vi "draw an ellipse.vi"(4 "ellipse factor":dbl=10.0, 6 "number of points":i32=20, 8 "curvature tensor IN":T3={"curvature Matrix"=[[3.0, 1.0], [1.0, 4.0]], "Eigenvalues"=[], "Eigenvectors"=[], "theta (rad)"=0.0+0.0i, "theta (deg)"=0.0+0.0i}, 10 "curvature Matrix IN":T1, 11 "center IN":cluster{"center x":dbl, "center Y":dbl}) -> (0 "curvature tensor OUT":T3={"curvature Matrix"=[[3.0, 1.0], [1.0, 4.0]], "Eigenvalues"=[4.618033988749895+0.0i, 2.381966011250105+0.0i], "Eigenvectors"=[[-0.8506508083520399+0.0i, -0.5257311121191335+0.0i], [0.5257311121191335+0.0i, -0.8506508083520399+0.0i]], "theta (rad)"=0.5535743588970453+0.0i, "theta (deg)"=31.717474411461012+0.0i}, 2 "curvature Matrix OUT":T1=[[3.0, 1.0], [1.0, 4.0]], 3 "ellipse OUT":cluster{"Array":dbl[], "Array":dbl[]})   [LabVIEW 2020]
uses:
  <vilib>/Analysis/Matrix/Datatypes/RealMatrix.ctl
  <vilib>/Analysis/Matrix/Datatypes/ComplexMatrix.ctl
  <vilib>/Analysis/7linalg.llb/Eigenvalue and Vectors Output Option.ctl
  array -- bilinear regression 2D.ctl
  <vilib>/Analysis/coordinate.llb/2D Cartesian Coordinate Rotation (Array).vi
  generate linear region.vi
  <vilib>/Analysis/7linalg.llb/Real Eigenvalues and Vectors.vi
  <vilib>/Analysis/Matrix/Numeric/Conversions/Matrix To Array - CM.vi
  <vilib>/Analysis/NI_AALPro.lvlib
  <vilib>/Analysis/Matrix/NI_Matrix.lvlib
panel:
  out "angle1":dbl=2.1243706856919418
  out "Plot: curvature":cluster{dbl[], dbl[]}(graph)
  out "z out":dbl[](array[numeric])
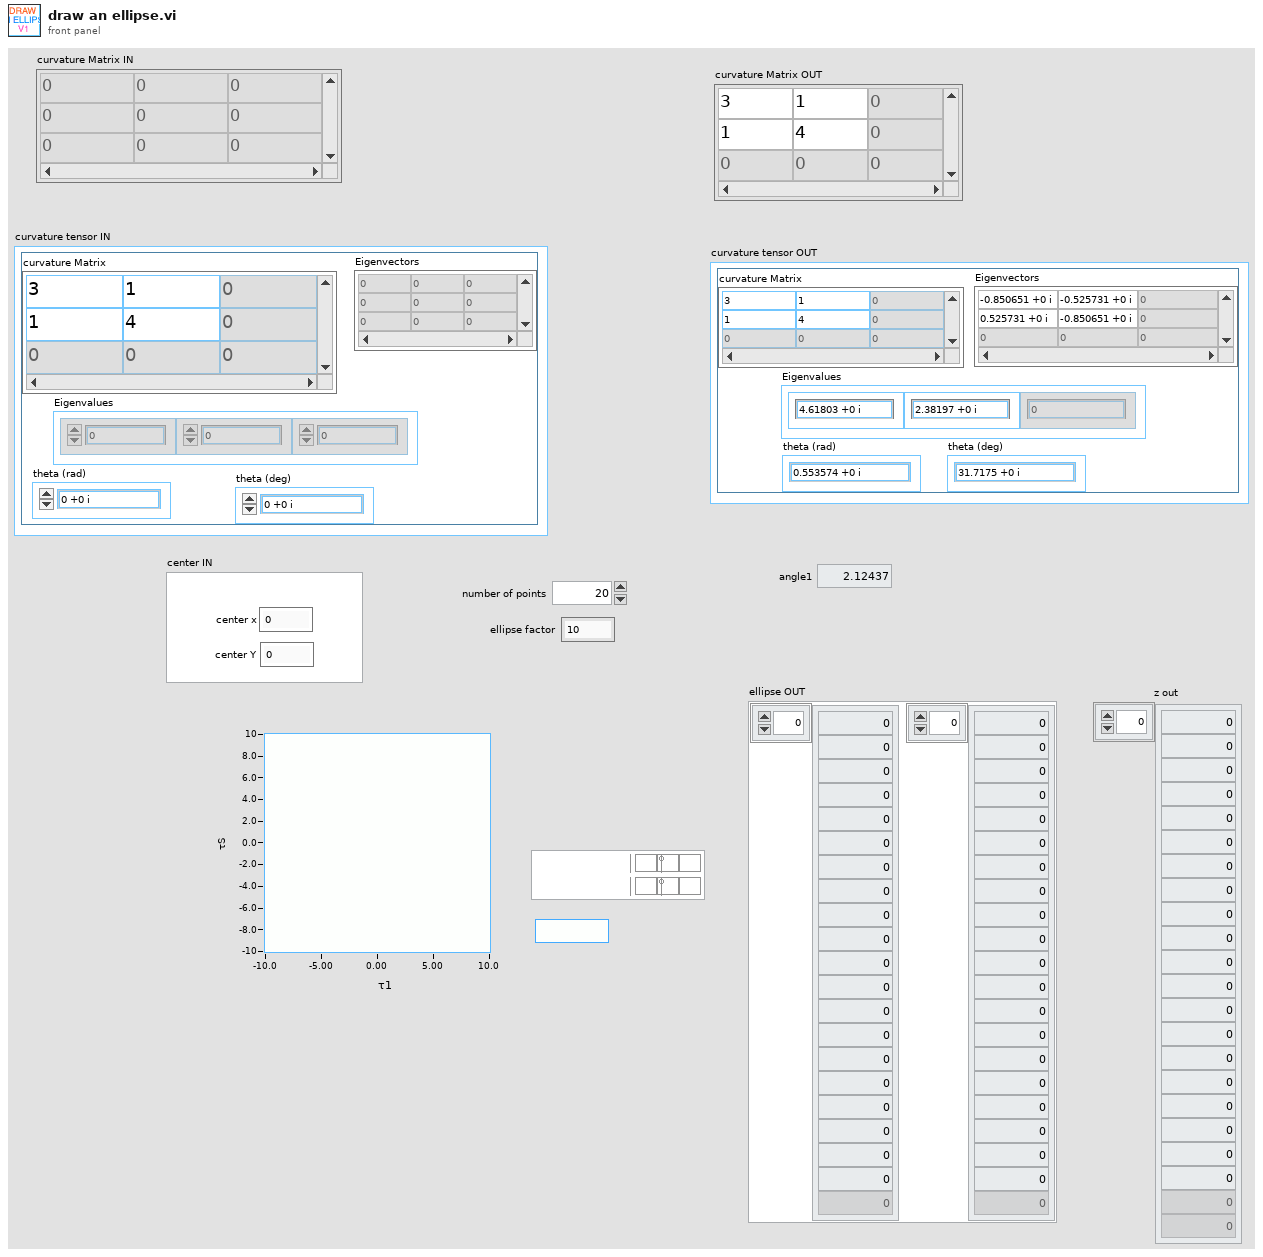
[diagram p1: front panel]
types:
  T1 = typedef "NI_Matrix.lvlib/RealMatrix.ctl" = dbl[][]
  T2 = typedef "NI_Matrix.lvlib/ComplexMatrix.ctl" = cdb[][]
  T3 = cluster{"curvature Matrix":T1, "Eigenvalues":cdb[], "Eigenvectors":T2, "theta (rad)":cdb, "theta (deg)":cdb}
  T4 = typedef "array -- bilinear regression 2D.ctl" = enum16{"1", "x", "y", "xx", "xy", "yy", "xxy", "xyy", "yyy", "xxx", "xxyy", "xyyy", "xxxy", "yyyy", "xxxx", "xxz", "xyz", "yyz", "xz", "yz", "z"}
  T5 = typedef "NI_AALPro.lvlib/Eigenvalue and Vectors Output Option.ctl" = i32
  T6 = cluster{"curvature Matrix":T1, dbl[], "Eigenvectors":T2, dbl, dbl}
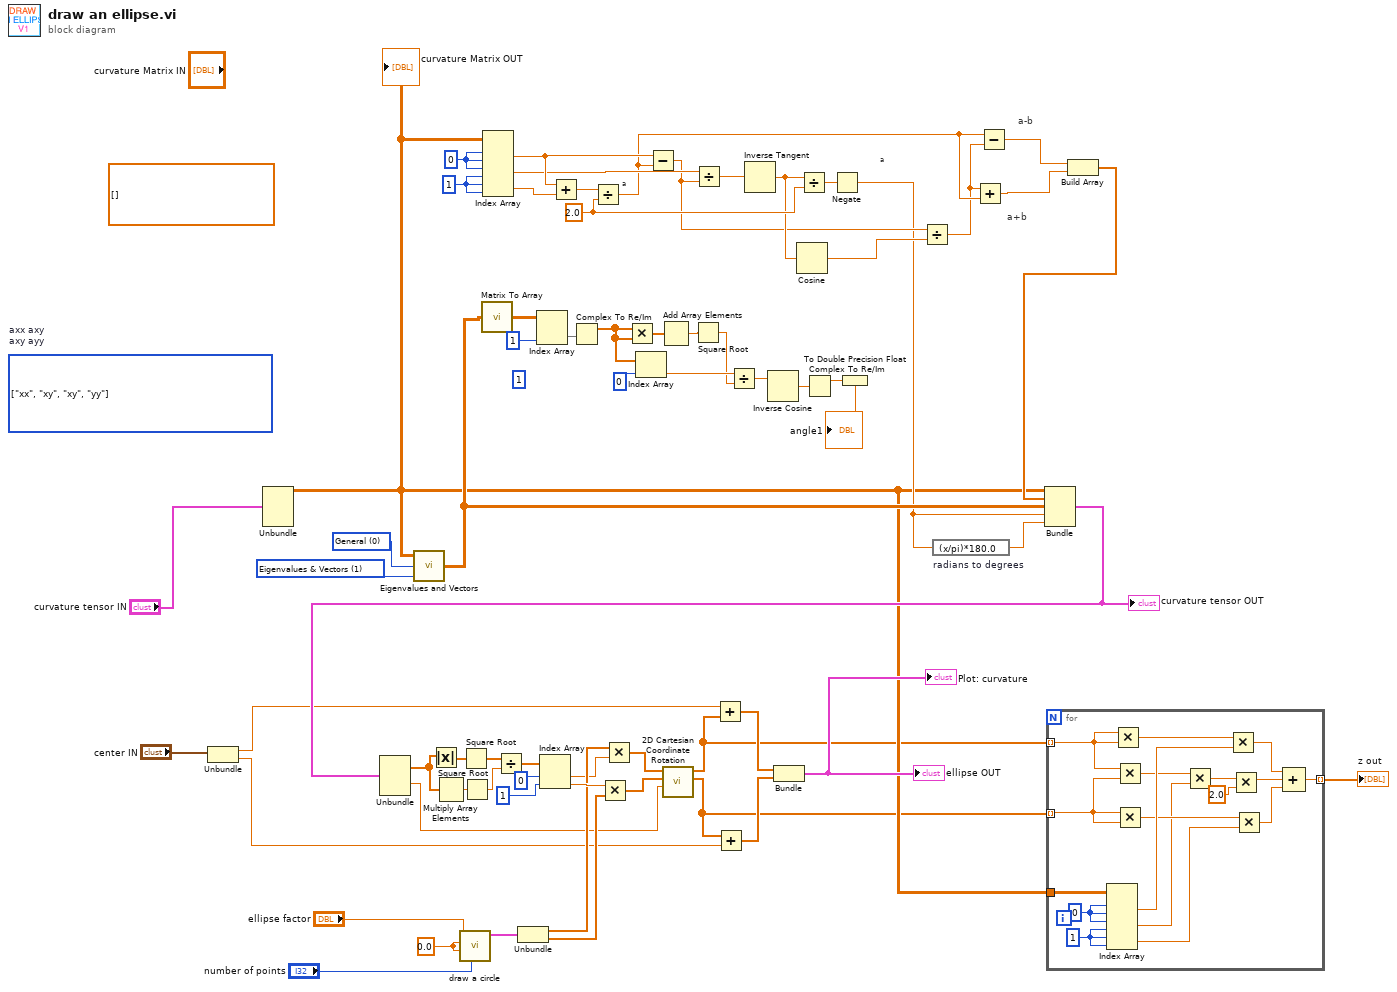
[diagram p0: block diagram]
diagram:
  (unwired) T1 [] ("curvature Matrix IN")
  w25 = 2.0 ("y")
  w30 = 1 ("index (row)")
  w31 = 0 ("index (row)")
  (unwired) T4[][] [[enum."xx", enum."xy"], [enum."xy", enum."yy"]] items=["1", "x", "y", "xx", "xy", "yy", "xxy", "xyy", "yyy", "xxx", "xxyy", "xyyy", "xxxy", "yyyy", "xxxx", "xxz", "xyz", "yyz", "xz", "yz", "z"]  # axx axy axy ayy
  (unwired) 1 ("length")
  w55 = T5 1 items=["Eigenvalues", "Eigenvalues & Vectors"] ("output option")
  w54 = 0 items=["General", "Symmetric"] ("matrix type")
  w58 = 0.0 ("center x")
  # "a-b"
  # "a+b"
  # "a"
  # "a"
  n1 = Unbundle("center IN") -> ("center x"=w4:dbl, "center Y"=w3:dbl)
  n2 = Unbundle("curvature tensor IN") -> ("curvature Matrix"=w8:T1)  [unwired: 4 out]
  "curvature Matrix OUT" <- w8
  n3 = call-poly <vilib>:"Eigenvalues and Vectors.vi"("output option"=w55, "matrix type"=w54, "Input Matrix"=w8) -> ("Eigenvectors"=w47:T2)  [unwired: 2 out]
  n4 = call "draw a circle.vi"("number of points"="number of points", "center Y"=w58, "center x"=w58, "radius"="ellipse factor") -> ("output cluster"=w65:cluster{dbl[], dbl[]})  [unwired: 7 in]
  n5 = call-poly <vilib>:"Matrix To Array.vi"("Complex Matrix"=w47) -> ("Complex 2D Array"=w46:cdb[][])
  n6 = Index Array(array=w8, index (row) #1=w31, index (col) #1=w31, index (row) #2=w31, index (col) #2=w30, index (row) #3=w30, index (col) #3=w30) -> (element #1=w27:dbl, element #2=w23:dbl, element #3=w29:dbl)
  n7 = Unbundle(w65) -> (w34:dbl[], w64:dbl[])
  n8 = Index Array(array=w46, index (col)=1 ("disabled index (col)")) -> (element=w44:cdb[])  [unwired: 1 in]
  n9 = Add(x=w27, y=w29) -> (x+y=w28:dbl)
  n10 = Complex To Re/Im(x + iy=w44) -> (x=w43:dbl[])  [unwired: 1 out]
  n11 = Divide(x=w28, y=w25) -> (x/y=w19:dbl)
  n12 = Multiply(x=w43, y=w43) -> (x*y=w52:dbl[])
  n13 = Index Array(array=w43, index=0 ("disabled index (col)")) -> (element=w50:dbl)
  n14 = Subtract(x=w27, y=w19) -> (x-y=w21:dbl)
  n15 = Add Array Elements(numeric array=w52) -> (sum=w45:dbl)
  n16 = Square Root(x=w45) -> (sqrt(x)=w49:dbl)
  n17 = Divide(x=w23, y=w21) -> (x/y=w26:dbl)
  n18 = Divide(x=w50, y=w49) -> (x/y=w48:dbl)
  n19 = Inverse Tangent(1:w26) -> (0:w22:dbl)
  n20 = Inverse Cosine(1:w48) -> (0:w42:dbl)
  n21 = Cosine(x=w22) -> (cos(x)=w20:dbl)
  n22 = Divide(x=w22, y=w25) -> (x/y=w24:dbl)
  n23 = Complex To Re/Im(x + iy=w42) -> (x=w41:dbl)  [unwired: 1 out]
  n24 = Negate(x=w24) -> (-x=w16:dbl)
  n25 = To Double Precision Float(number=w41) -> (double precision float=→"angle1":dbl)
  n26 = Divide(x=w21, y=w20) -> (x/y=w18:dbl)
  n27 = expression code="(x/pi)*180.0" "radians to degrees"(w16) -> (w39:dbl)
  n28 = Add(x=w18, y=w19) -> (x+y=w13:dbl)
  n29 = Subtract(x=w19, y=w18) -> (x-y=w14:dbl)
  n30 = Build Array(w14, w13) -> (w17:dbl[])
  n31 = Bundle("curvature Matrix"=w8, w17, "Eigenvectors"=w47, w16, w39) -> (w40:T6)  [unwired: 1 in]
  "curvature tensor OUT" <- w40
  n32 = Unbundle(w40) -> (w2:dbl[], w32:dbl)  [unwired: 3 out]
  n33 = Absolute Value(x=w2) -> (abs(x)=w56:dbl[])
  n34 = Multiply Array Elements(1:w2) -> (0:w12:dbl)
  n35 = Square Root ("Square Root.vi")(x=w56) -> (sqrt(x)=w11:dbl[])
  n36 = Square Root(x=w12) -> (sqrt(x)=w1:dbl)
  n37 = Divide(x=w11, y=w1) -> (x/y=w10:dbl[])
  n38 = Index Array(array=w10, index #1=0 ("index"), index #2=1 ("index")) -> (element #1=w33:dbl, element #2=w61:dbl)
  n39 = Multiply(x=w61, y=w64) -> (x*y=w59:dbl[])
  n40 = Multiply(x=w34, y=w33) -> (x*y=w60:dbl[])
  n41 = call-poly <vilib>:"2D Cartesian Coordinate Rotation.vi"("theta"=w32, "Y"=w59, "X"=w60) -> ("Y Out"=w6:dbl[], "X Out"=w7:dbl[])  [unwired: 6 in, 1 out]
  n42 = Add(x=w4, y=w7) -> (x+y=w38:dbl[])
  n43 = Add(x=w6, y=w3) -> (x+y=w37:dbl[])
  n44 = Bundle(w38, w37) -> (→"ellipse OUT" →"Plot: curvature":cluster{dbl[], dbl[]})  [unwired: 1 in]
  n45 = for {
    tunnel: w7 -> [w80] mode=indexing
    tunnel: w6 -> [w79] mode=indexing
    tunnel: w8 -> [w83]
    tunnel: [w67] -> w36 mode=indexing
    w81 = 1 ("index (row)")
    w82 = 0 ("index (row)")
    n46 = Index Array(array=w83, index (row) #1=w82, index (col) #1=w82, index (row) #2=w82, index (col) #2=w81, index (row) #3=w81, index (col) #3=w81) -> (element #1=w77:dbl, element #2=w74:dbl, element #3=w76:dbl)
    n47 = Multiply(x=w80, y=w80) -> (x*y=w78:dbl)
    n48 = Multiply(x=w80, y=w79) -> (x*y=w73:dbl)
    n49 = Multiply(x=w79, y=w79) -> (x*y=w75:dbl)
    n50 = Multiply(x=w73, y=w74) -> (x*y=w72:dbl)
    n51 = Multiply(x=w78, y=w77) -> (x*y=w70:dbl)
    n52 = Multiply(x=w72, y=2.0) -> (x*y=w69:dbl)
    n53 = Multiply(x=w75, y=w76) -> (x*y=w68:dbl)
    n54 = Compound Arithmetic op=ADD(w70, w69, w68) -> (w67:dbl)
  }
  "z out" <- w36
